vi "Result_Test.vi"(8 "error in (no error)":errorcluster caption="entrée d'erreur (pas d'erreur)", 11 "Flash_Jlink en entrée":refnum<class "FW_Check_Hash_code.lvclass">) -> (0 "error out":errorcluster caption="sortie d'erreur", 3 "Flash_Jlink en sortie":refnum<class "FW_Check_Hash_code.lvclass">)   [LabVIEW 2020, in "Library Test.lvlib" / "FW_Check_Hash_code.lvclass"]
uses:
  FW_Check_Hash_code.lvclass
  C:/Users/ngarcin/OneDrive - Altyor/Standard TB/Class/Test/Test (Default)/Test (Default).lvclass
  Test_Without_Instr/Test_Without_Inst.lvclass
  FW_Check_Hash_code.lvclass/FW_Check_Hash_code.ctl
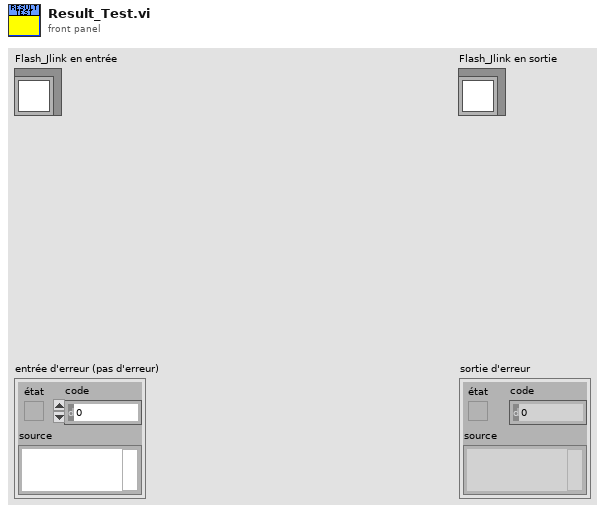
[diagram p1: front panel]
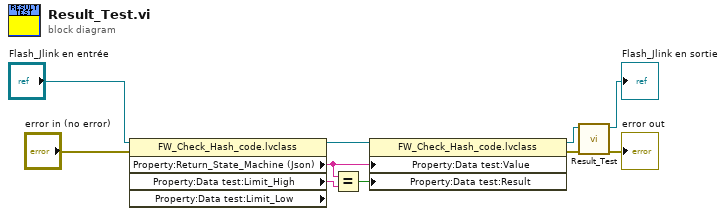
[diagram p0: block diagram]
diagram:
  n1 = property class="FW_Check_Hash_code.lvclass" props=["Property:Return_State_Machine (Json)", "Property:Data test:Limit_High", "Property:Data test:Limit_Low"](reference="Flash_Jlink en entrée", error in="error in (no error)") -> (reference out=w5:refnum<class "FW_Check_Hash_code.lvclass">, "Property:Return_State_Machine (Json)"=w1:string, "Property:Data test:Limit_High"=w3:string)  [unwired: 2 out]
  n2 = Equal?(x=w1, y=w3) -> (x = y?=w2:bool)
  n3 = property class="FW_Check_Hash_code.lvclass"(reference=w5, "Property:Data test:Value"=w1, "Property:Data test:Result"=w2) -> (reference out=w4:refnum<class "FW_Check_Hash_code.lvclass">, error out=w8:errorcluster)  [unwired: 1 in]
  n4 = call-parent "Result_Test.vi"("error in (no error)"=w8, "Test_Without_Inst en entrée"=w4) -> ("error out"=→"error out":errorcluster, "Test_Without_Inst en sortie"=→"Flash_Jlink en sortie":refnum<class "FW_Check_Hash_code.lvclass">)  [unwired: 8 in]
